vi "Parse String.vi"(8 "Error In":errorcluster, 9 "JSON Response":string, 10 "Key":string, 11 "XBMC Ref":T1={"HTTP Handle"=refnum, "Hostname / IP"="localhost", "jsonrpc"="2.0"}) -> (0 "Error Out":errorcluster, 1 "Dup JSON Response":string, 2 "Value":string, 3 "XBMC Ref":T1={"HTTP Handle"=refnum, "Hostname / IP"="localhost", "jsonrpc"="2.0"})   [LabVIEW 2013, in "LVH-XBMC.lvlib"]
uses:
  LVH-XBMC.lvlib
  Type Defs/XBMC Ref.ctl
  <vilib>/httpClient/ClientHandle.ctl
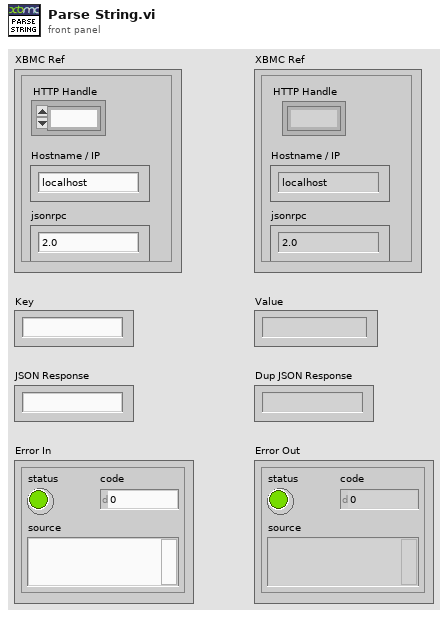
[diagram p1: front panel]
types:
  T1 = typedef "LVH-XBMC.lvlib/XBMC Ref.ctl" = cluster{"HTTP Handle":T2, "Hostname / IP":string, "jsonrpc":string}
  T2 = typedef "LabVIEWHTTPClient.lvlib/ClientHandle.ctl" = refnum<k1>
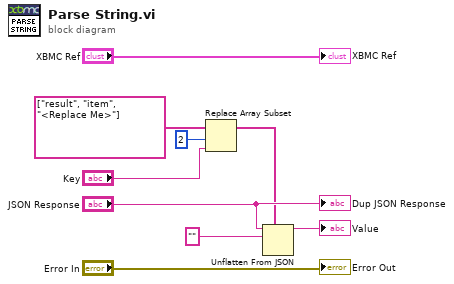
[diagram p0: block diagram]
diagram:
  n1 = Replace Array Subset(array=string[] ["result", "item", "<Replace Me>"] ("path"), new element="Key", index=2) -> (w4:string[])
  n2 = Unflatten From JSON(path=w4, JSON string="JSON Response", type and defaults="") -> (value=→"Value":string)  [unwired: 4 in, 1 out]
  "Dup JSON Response" <- "JSON Response"
  "Error Out" <- "Error In"
  "XBMC Ref" <- "XBMC Ref"
